vi "Read Config Data.vi"(8 "error in (no error)":errorcluster, 11 "Sequence Builder in":refnum<class "Sequence Builder.lvclass">) -> (0 "error out":errorcluster, 2 "Config Data":refnum<class "Data.lvclass">[](array[class]), 3 "Sequence Builder out":refnum<class "Sequence Builder.lvclass">)   [LabVIEW 2015, in "Sequence Composition.lvlib" / "Sequence Builder.lvclass"]
uses:
  Sequence Builder.lvclass
  Data/Data.lvclass
  Sequence Builder.lvclass/Sequence Builder.ctl
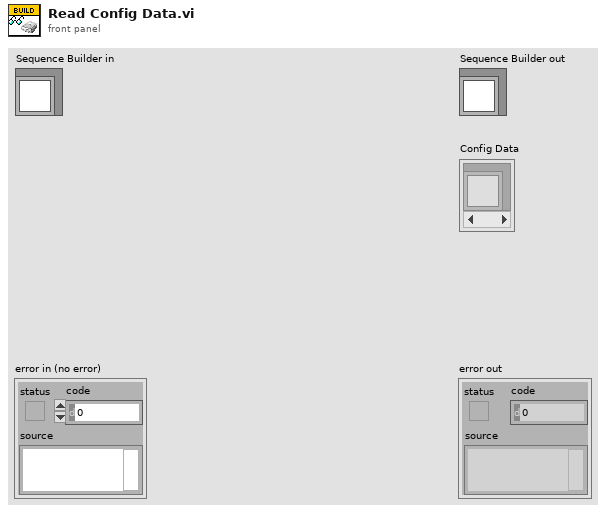
[diagram p1: front panel]
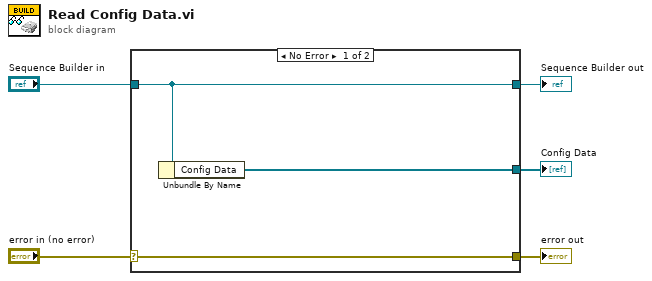
[diagram p0: block diagram]
diagram:
  n1 = case shown="No Error" "error in (no error)" {
    selector: "error in (no error)" -> [w8 w9]
    tunnel: [w8 w9] -> w4
    tunnel: [w7 w10] -> w2
    tunnel: "Sequence Builder in" -> [w7 w10]
    tunnel: [w6 _] -> w1
    frame No Error {
      n2 = Unbundle By Name(w7) -> ("Config Data"=w6:refnum<class "Data.lvclass">[])
    }
    frame Error {
    }
  }
  "error out" <- w4
  "Sequence Builder out" <- w2
  "Config Data" <- w1
